vi "get Userinfo List.vi"(2 "userinfo list":T1, 8 "error in (no error)":errorcluster, 11 "[User] Userinfo Binary in":refnum<class "[User] Userinfo Binary.lvclass">) -> (0 "error out":errorcluster, 3 "[User] Userinfo Binary out":refnum<class "[User] Userinfo Binary.lvclass">)   [LabVIEW 2020, in "[User] Userinfo Binary.lvclass"]
uses:
  [User] Userinfo Binary.lvclass
  [User] Userinfo/Control/userinfo list.ctl
  [User] Userinfo/[User] Userinfo.lvclass
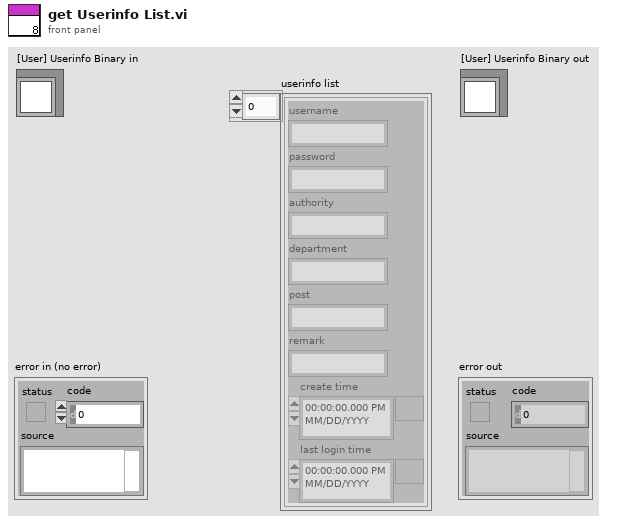
[diagram p1: front panel]
types:
  T1 = typedef "[User] Userinfo.lvclass/userinfo list.ctl" = cluster{"username":string, "password":string, "authority":string, "department":string, "post":string, "remark":string, "create time":timestamp, "last login time":timestamp}[]
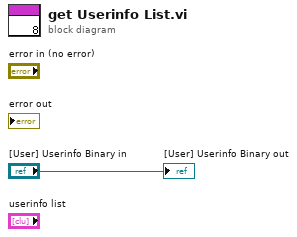
[diagram p0: block diagram]
diagram:
  "[User] Userinfo Binary out" <- "[User] Userinfo Binary in"
